vi "M07 Solar Cells.vi"(9 "Target angle":sgl, 11 "EV3 in":T1) -> (3 "EV3 out":T1)   [LabVIEW 2016]
uses:
  <vilib>/NXT/Subs/LVHSConnector.ctl
  <vilib>/NXT/LegoClasses/BrickReference/BrickReference.lvclass
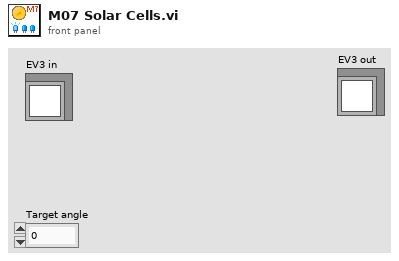
[diagram p1: front panel]
types:
  T1 = typedef "LVHSConnector.ctl" = refnum<class "BrickReference.lvclass">
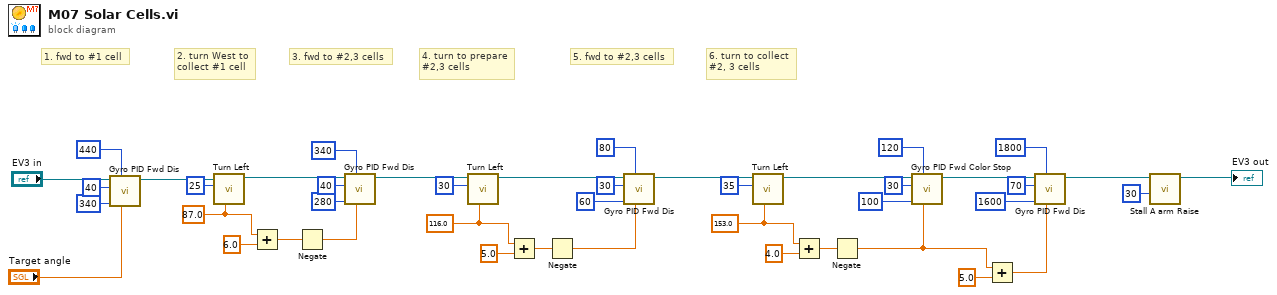
[diagram p0: block diagram]
diagram:
  w16 = sgl 153.0 ("Turning angle")
  w24 = sgl 116.0 ("Turning angle")
  w40 = sgl 87.0 ("Turning angle")
  # "6. turn to collect\n#2, 3 cells"
  # "5. fwd to #2,3 cells"
  # "4. turn to prepare\n#2,3 cells"
  # "3. fwd to #2,3 cells"
  # "2. turn West to\ncollect #1 cell"
  # "1. fwd to #1 cell"
  n1 = call "Gyro PID Fwd Dis.vi"("Target angle"="Target angle", "Threshold to stop"=440, "Threshold to slow"=340, "Max. speed"=40, "EV3 in"="EV3 in") -> ("EV3 out"=w37:T1)  [unwired: 6 in]
  n2 = call "Turn Left.vi"("Turning angle"=w40, "Motor B (right)"=i8 25, "EV3 in"=w37) -> ("EV3 out"=w33:T1)  [unwired: 8 in]
  n3 = Add(x=w40, y=sgl 6.0) -> (x+y=w38:sgl)
  n4 = Negate(x=w38) -> (-x=w32:sgl)
  n5 = call "Gyro PID Fwd Dis.vi"("Target angle"=w32, "Threshold to stop"=340, "Threshold to slow"=280, "Max. speed"=40, "EV3 in"=w33) -> ("EV3 out"=w30:T1)  [unwired: 6 in]
  n6 = call "Turn Left.vi"("Turning angle"=w24, "Motor B (right)"=i8 30, "EV3 in"=w30) -> ("EV3 out"=w29:T1)  [unwired: 8 in]
  n7 = Add(x=w24, y=sgl 5.0) -> (x+y=w26:sgl)
  n8 = Negate(x=w26) -> (-x=w21:sgl)
  n9 = call "Gyro PID Fwd Dis.vi"("Target angle"=w21, "Threshold to stop"=80, "Threshold to slow"=60, "Max. speed"=30, "EV3 in"=w29) -> ("EV3 out"=w11:T1)  [unwired: 6 in]
  n10 = call "Turn Left.vi"("Turning angle"=w16, "Motor B (right)"=i8 35, "EV3 in"=w11) -> ("EV3 out"=w13:T1)  [unwired: 8 in]
  n11 = Add(x=w16, y=sgl 4.0) -> (x+y=w14:sgl)
  n12 = Negate(x=w14) -> (-x=w6:sgl)
  n13 = call "Gyro PID Fwd Color Stop.vi"("Target angle"=w6, "Threshold to Color"=120 ("Threshold to stop"), "Threshold to slow"=100, "Max. speed"=30, "EV3 in"=w13) -> ("EV3 out"=w10:T1)  [unwired: 6 in]
  n14 = Add(x=w6, y=sgl 5.0) -> (x+y=w4:sgl)
  n15 = call "Gyro PID Fwd Dis.vi"("Target angle"=w4, "Threshold to stop"=1800, "Threshold to slow"=1600, "Max. speed"=70, "EV3 in"=w10) -> ("EV3 out"=w3:T1)  [unwired: 6 in]
  n16 = call "Stall A arm Raise.vi"("Power"=i8 30, "NXT/EV3"=w3) -> ("NXT/EV3"=→"EV3 out":T1)  [unwired: 9 in]
